vi "plot all temp channels differential.vi"() -> ()   [LabVIEW 2011]
uses:
  <vilib>/Utility/error.llb/DialogType.ctl
  <vilib>/DAQmx/read.llb/DAQmx Read (Analog 2D DBL NChan NSamp).vi
  <vilib>/Utility/file.llb/Write To Spreadsheet File (DBL).vi
  <vilib>/DAQmx/miscellaneous.llb/DAQmx Fill In Error Info.vi
  <vilib>/Analysis/NI_AALBase.lvlib
panel:
  in  "DAQmx Task Name":refnum<k21>
  out "Waveform Chart 2":T1(graph)
  in  "temp sensor channels":tag="Dev3/ai0:3"
  in  "stop":bool
  in  "error in":errorcluster
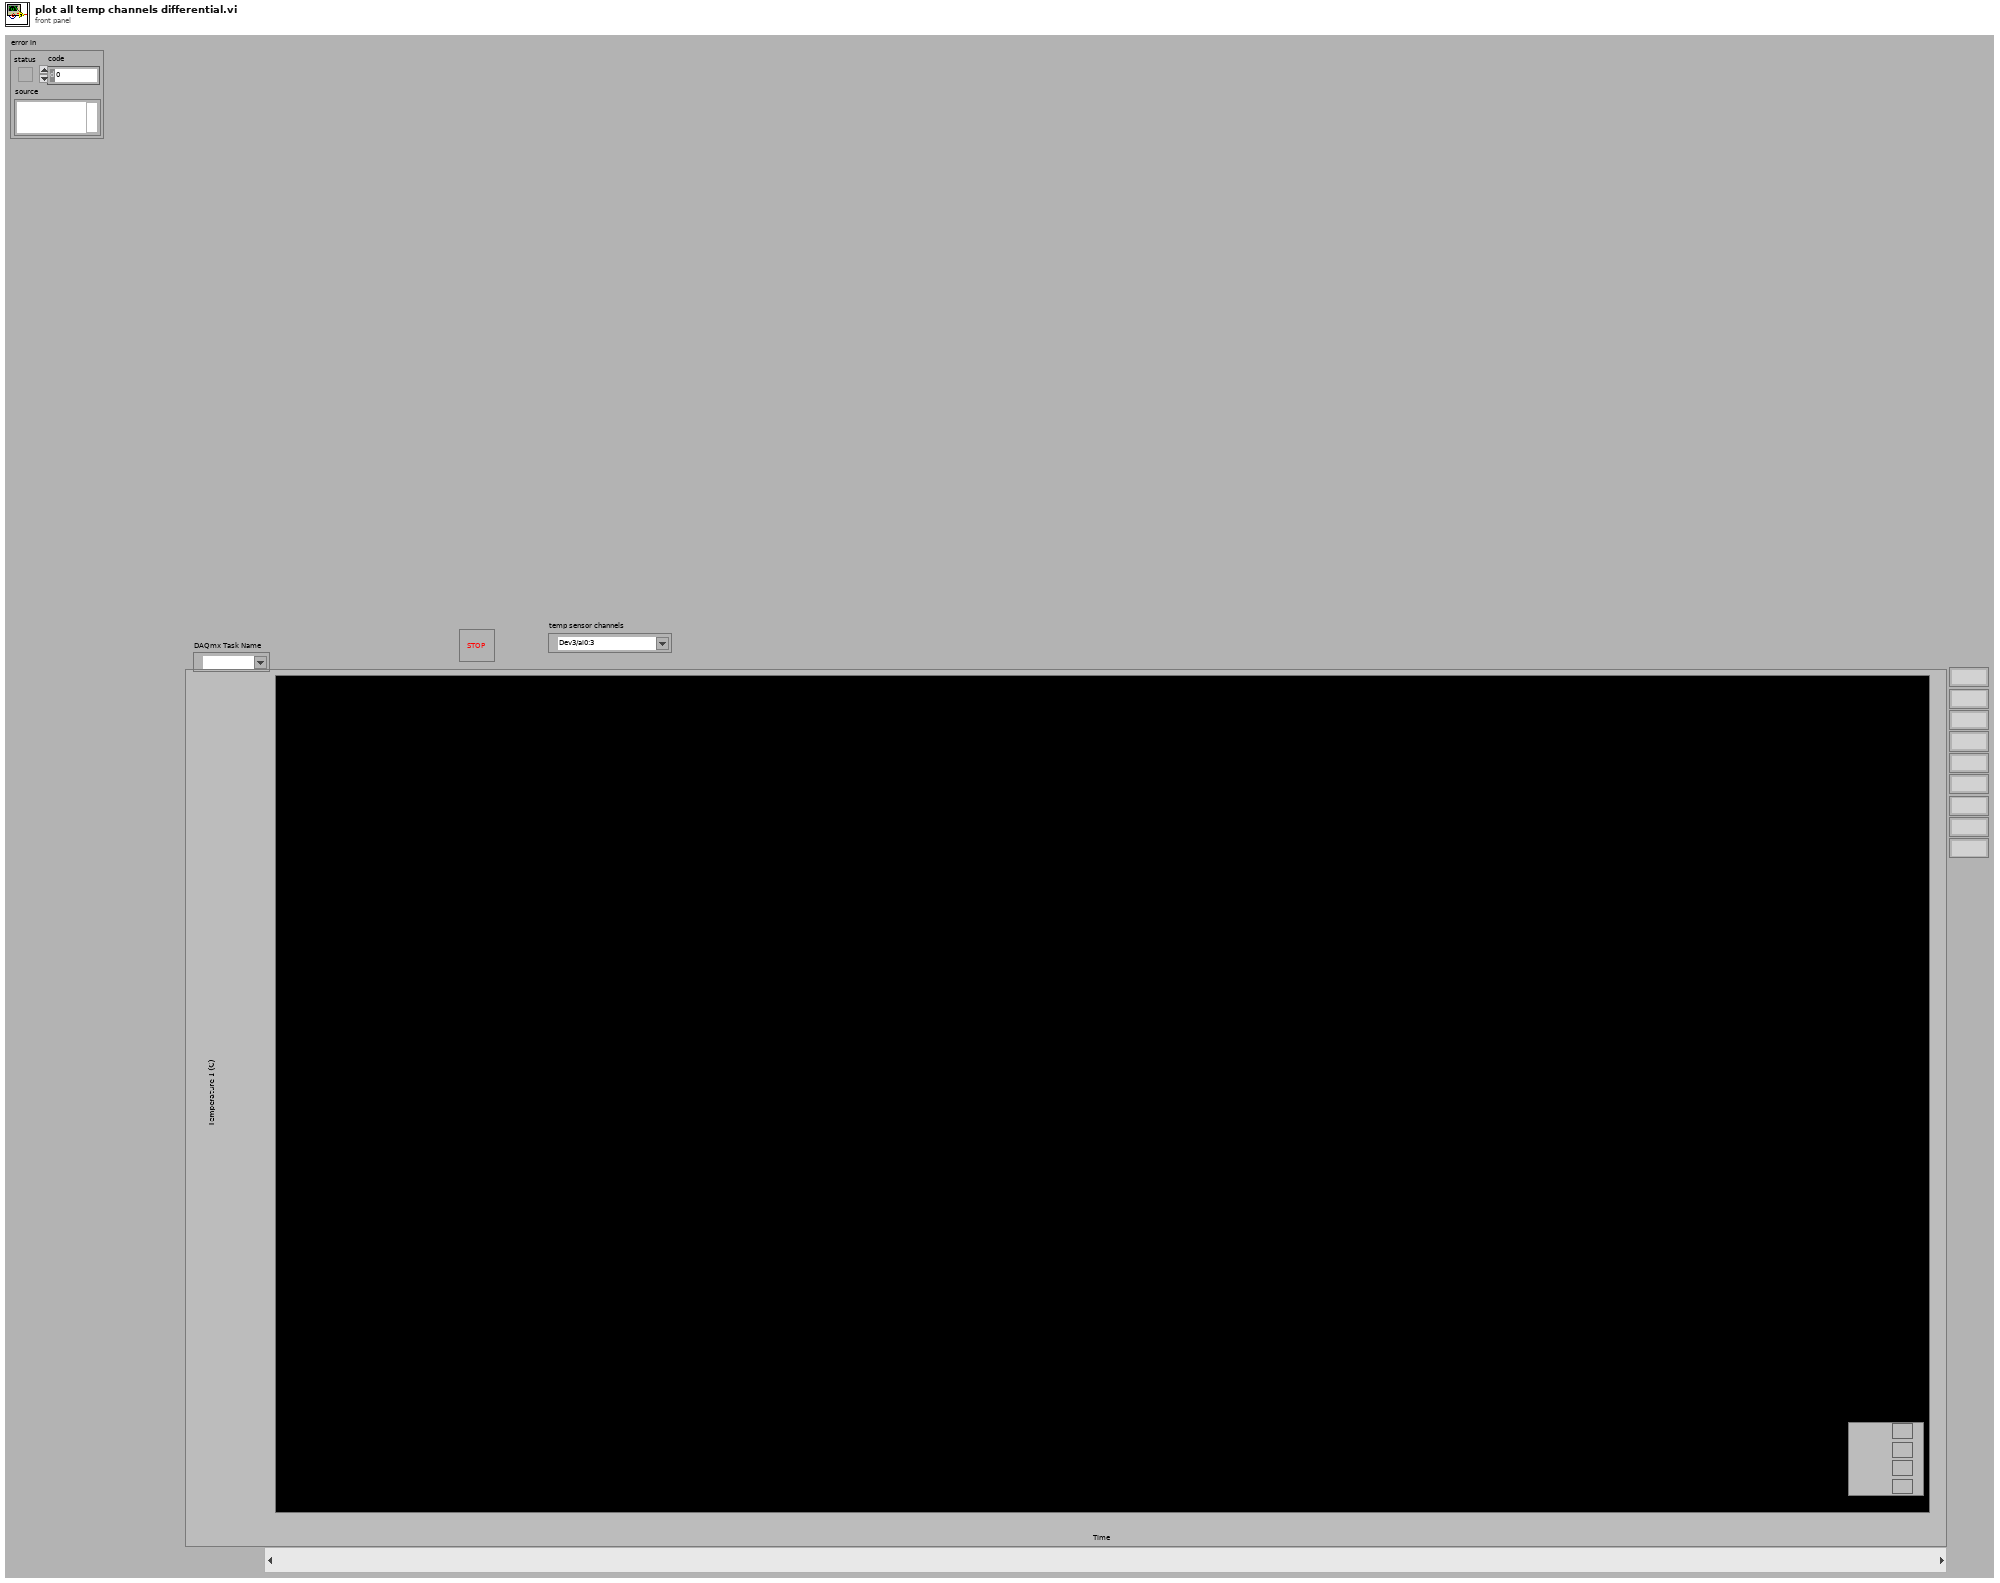
[diagram p1: front panel]
types:
  T1 = cluster{"[0]":dbl, "[1]":dbl, "[2]":dbl, "[3]":dbl, "[4]":dbl, "[5]":dbl, "[6]":dbl, "[7]":dbl, "[8]":dbl}
  T2 = typedef "DialogType.ctl" = u16
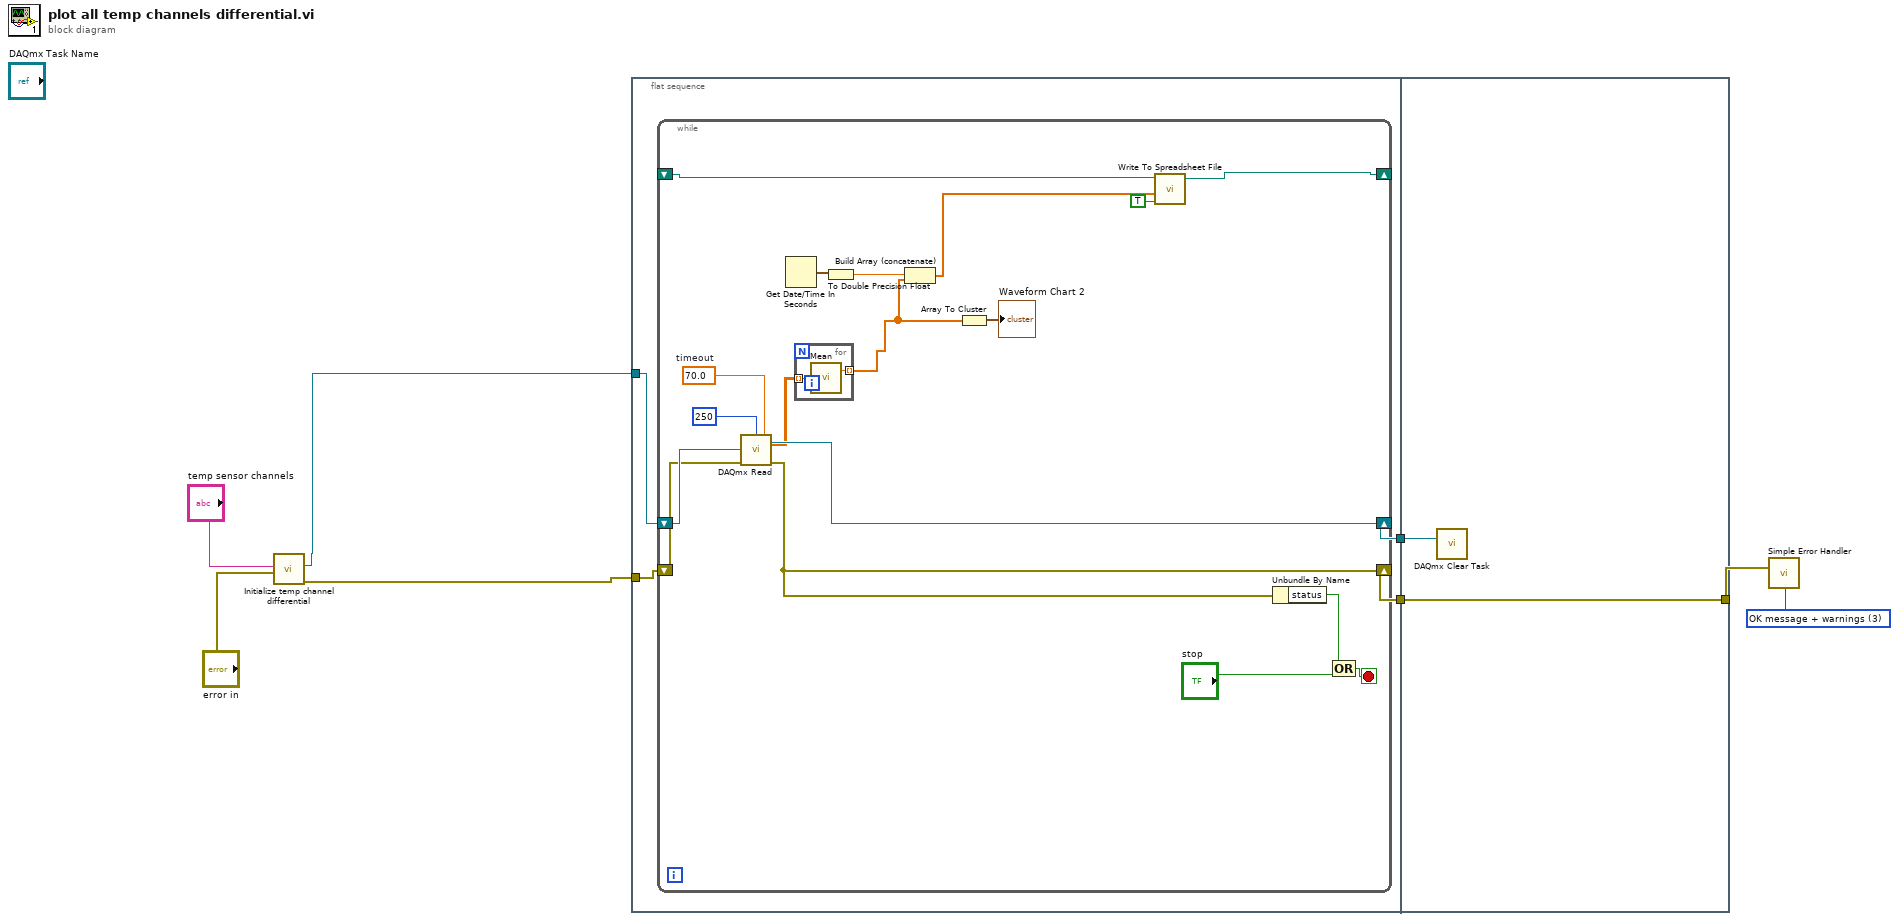
[diagram p0: block diagram]
diagram:
  w7 = T2 3 items=["no dialog", "OK message", "continue or stop message", "OK message + warnings", "continue/stop + warnings"] ("type of dialog (OK msg:1)")
  n1 = call "Initialize temp channel differential.vi"("error in"="error in", "Physical channel"="temp sensor channels") -> ("error out"=w1:errorcluster, "task out"=w2:refnum<k21>)  [unwired: 6 out]
  n2 = flat-sequence {
    tunnel: w2 -> [w12]
    tunnel: [w11] -> w6
    tunnel: [w10] -> w5
    tunnel: w1 -> [w9]
    tunnel: [w34] -> w8
    tunnel: w6 -> [w33]
    tunnel: w5 -> [w34]
    frame #0 {
      n3 = while {
        shift-right: [w13] -> w10
        shift-left: w9 -> [w27]
        shift-right: [w26] -> w11
        shift-left: w12 -> [w28]
        shift-right: [w17] -> _
        shift-left: _ -> [w16]
        stop <- w29 stop-if-true
        w25 = 70.0  # timeout
        n4 = call-poly <vilib>:"DAQmx Read.vi"("task/channels in"=w28, "number of samples per channel"=250, "timeout"=w25, "error in"=w27) -> ("task out"=w26:refnum<k21>, "data"=w23:dbl[][], "error out"=w13:errorcluster)  [unwired: 9 out]
        n5 = Get Date/Time In Seconds() -> (seconds since 1Jan1904=w22:timestamp)
        n6 = for {
          tunnel: [w32] -> w20 mode=indexing
          tunnel: w23 -> [w31] mode=indexing
          n7 = call <vilib>:"Mean.vi"("X"=w31) -> ("mean"=w32:dbl)  [unwired: 1 out]
        }
        n8 = To Double Precision Float(number=w22) -> (double precision float=w19:dbl)
        n9 = Build Array (concatenate)(w19, w20) -> (w15:dbl[])
        n10 = Array To Cluster(array=w20) -> (cluster=→"Waveform Chart 2":T1)
        n11 = call-poly <vilib>:"Write To Spreadsheet File.vi"("append to file? (new file:F)"=TRUE, "1D data"=w15, "file path (dialog if empty)"=w16) -> ("new file path (Not A Path if cancelled)"=w17:path)  [unwired: 5 in]
        n12 = Unbundle By Name(w13) -> ("status"=w18:bool)
        n13 = Compound Arithmetic op=OR(w18, "stop") -> (w29:bool)
      }
    }
    frame #1 {
      n14 = call <vilib>:"DAQmx Clear Task.vi"("task in"=w33) -> ()  [unwired: 1 in, 14 out]
    }
  }
  n15 = call <vilib>:"Simple Error Handler.vi"("type of dialog (OK msg:1)"=w7, "error in (no error)"=w8) -> ()  [unwired: 8 out]
